vi "RTS Check Chamber Conditions Send Command.vi"(8 "Error In":errorcluster, 10 "Chamber 1-1":T1 {"Start Time" format="%<%X\n%x>T"; "End Time" format="%<%X\n%x>T"}, 11 "Room Setpoints":T4 {"Room Dehum Temperature (*RM De Hum Set P1)" min=30.0 max=120.0; "Room Cool Temperature (*RM Cool Setp 1)" min=30.0 max=120.0; "Room Setpoint Humidity (*RM Hum Set P1)" min=5.0 max=98.0; "Room Setpoint Temperature (*RM Dry Set P1)" min=40.0 max=120.0}) -> (0 "Error Out":errorcluster, 2 "New Conditions":T1 {"Start Time" format="%<%X\n%x>T"; "End Time" format="%<%X\n%x>T"}, 3 "Matching Setpoints?":bool)   [LabVIEW 2016]
uses:
  Type Definitions/RTS Chamber Temperature Humidity Control.ctl
  Type Definitions/RTS Door Ops Client.ctl
  Type Definitions/RTS Door Opening Schedule.ctl
  Type Definitions/RTS Door Ops Sequence.ctl
panel:
  # "Chamber Conditions:"
  # "Chamber Conditions:"
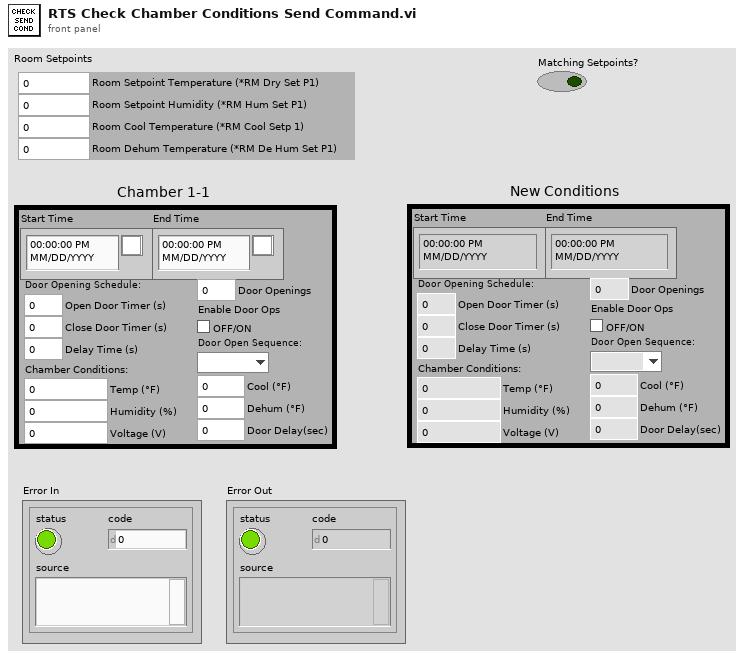
[diagram p1: front panel]
types:
  T1 = typedef "RTS Door Ops Client.ctl" = cluster{"End Time":timestamp, "Start Time":timestamp, "Door Opening Schedule:":T2, "Enable Door Ops":bool, "Door Openings":u32, "Temp (°F)":dbl, "Humidity (%)":dbl, "Voltage (V)":dbl, "Door Open Sequence:":T3, "Door Delay(sec)":dbl, "Dehum (°F)":dbl, "Cool (°F)":dbl}
  T2 = typedef "RTS Door Opening Schedule.ctl" = cluster{"Open Door Timer (s)":dbl, "Delay Time (s)":dbl, "Close Door Timer (s)":dbl}
  T3 = typedef "RTS Door Ops Sequence.ctl" = enum16{"", "1st", "2nd", "3rd"}
  T4 = typedef "RTS Chamber Temperature Humidity Control.ctl" = cluster{"Room Setpoint Temperature (*RM Dry Set P1)":dbl, "Room Setpoint Humidity (*RM Hum Set P1)":dbl, "Room Cool Temperature (*RM Cool Setp 1)":dbl, "Room Dehum Temperature (*RM De Hum Set P1)":dbl}
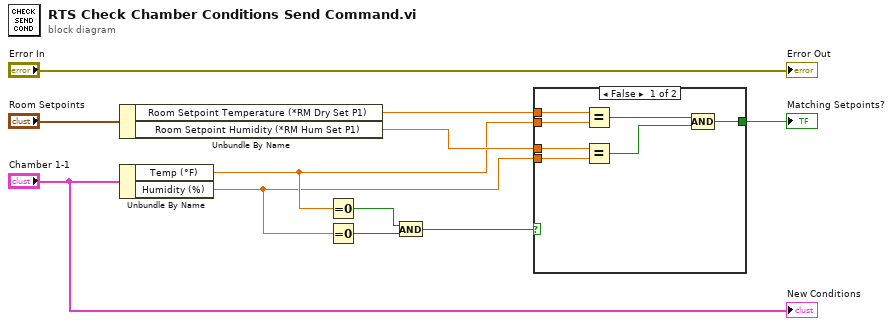
[diagram p0: block diagram]
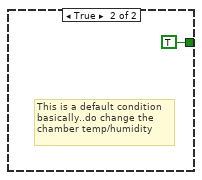
[diagram p2: hidden frame]
diagram:
  n1 = Unbundle By Name("Room Setpoints") -> ("Room Setpoint Temperature (*RM Dry Set P1)"=w9:dbl, "Room Setpoint Humidity (*RM Hum Set P1)"=w10:dbl)
  n2 = Unbundle By Name("Chamber 1-1") -> ("Temp (°F)"=w5:dbl, "Humidity (%)"=w4:dbl)
  n3 = Equal To 0?(x=w5) -> (x = 0?=w3:bool)
  n4 = Equal To 0?(x=w4) -> (x = 0?=w2:bool)
  n5 = And(x=w3, y=w2) -> (x .and. y?=w1:bool)
  n6 = case shown="False" w1 {
    tunnel: [w18 TRUE] -> w11
    tunnel: w10 -> [w15 _]
    tunnel: w9 -> [w14 _]
    tunnel: w5 -> [w13 _]
    tunnel: w4 -> [w12 _]
    frame False {
      n7 = Equal?(x=w14, y=w13) -> (x = y?=w16:bool)
      n8 = Equal?(x=w15, y=w12) -> (x = y?=w17:bool)
      n9 = Compound Arithmetic op=AND(w16, w17) -> (w18:bool)
    }
    frame True {
      # "This is a default condition\nbasically..do change the\nchamber temp/humidity"
    }
  }
  "Matching Setpoints?" <- w11
  "Error Out" <- "Error In"
  "New Conditions" <- "Chamber 1-1"
